vi "FrameInRange (SubVI).vi"(11 "Application in":refnum<vi>) -> (1 "in range":bool, 3 "Application ref out":refnum<vi>)   [LabVIEW 2014]
uses:
  <userlib>/Nanonis Prog Interface V5/Scan/Piezos/Piezo Calibration Range Get.vi
  <userlib>/Nanonis Prog Interface V5/Nanonis Prog Interface.lvlib
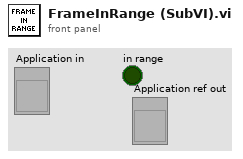
[diagram p1: front panel]
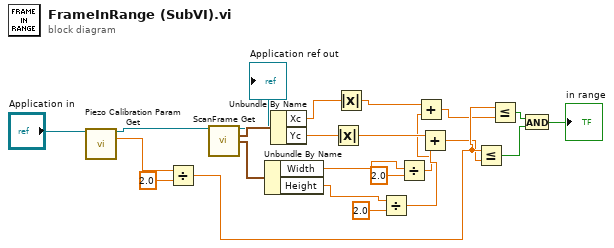
[diagram p0: block diagram]
diagram:
  n1 = call-poly <userlib>:"Piezo Calibration Param Get.vi"("Application ref in"="Application in") -> ("Application ref out"=w3:refnum<vi>, "Range X (m)"=w4:sgl)  [unwired: 10 in, 3 out]
  n2 = Divide(x=w4, y=sgl 2.0) -> (x/y=w20:sgl)
  n3 = call <userlib>:"ScanFrame Get.vi"("Application ref in"=w3) -> ("Application ref out"=→"Application ref out":refnum<vi>, "Center coordinates (m)"=w6:cluster{"Xc":sgl, "Yc":sgl}, "Size (m)"=w7:cluster{"Width":sgl, "Height":sgl})  [unwired: 10 in, 2 out]
  n4 = Unbundle By Name(w7) -> ("Width"=w12:sgl, "Height"=w13:sgl)
  n5 = Unbundle By Name(w6) -> ("Xc"=w8:sgl, "Yc"=w9:sgl)
  n6 = Absolute Value(x=w9) -> (abs(x)=w17:sgl)
  n7 = Absolute Value(x=w8) -> (abs(x)=w16:sgl)
  n8 = Divide(x=w13, y=sgl 2.0) -> (x/y=w15:sgl)
  n9 = Divide(x=w12, y=sgl 2.0) -> (x/y=w14:sgl)
  n10 = Add(x=w16, y=w14) -> (x+y=w18:sgl)
  n11 = Add(x=w17, y=w15) -> (x+y=w19:sgl)
  n12 = Less Or Equal?(x=w20, y=w19) -> (x <= y?=w22:bool)
  n13 = Less Or Equal?(x=w20, y=w18) -> (x <= y?=w21:bool)
  n14 = And(x=w21, y=w22) -> (x .and. y?=→"in range":bool)
